vi "LoL Chat Front.vi"() -> ()   [LabVIEW 2011]
uses:
  <vilib>/addons/database/Connection.llb/DB Tools Open Connec (Path).vi
  <vilib>/addons/database/Connection.llb/Conn Execute.vi
  <vilib>/addons/database/Recordset.llb/Rec Fetch Recordset Data (R).vi
  <vilib>/Utility/file.llb/Write To Spreadsheet File (string).vi
  <vilib>/addons/database/NI_Database_API.lvlib
panel:
  out "Waveform Chart":i32[](graph)
  in  "Chat Time (minutes)":cluster{dbl, dbl}(slide)={0.0, 62.22222086588542} scale=0.0..150.0
  in  "Game Length (minutes)":cluster{dbl, dbl}(slide)={0.0, 62.22222086588542} scale=0.0..150.0
  in  "Word Length":cluster{dbl, dbl}(slide)={0.0, 8.585858585858587} scale=0.0..20.0
  out "Sorted Word Frequencies":string[][](array[string])
  in  "Save Results":bool
  out "SQL Query Command":string
  in  "Number of Entries":string="1000"
  in  "Game Outcome":string(combo)="Victory"
  in  "Scrollbar":i32(c297)
  in  "Tab Control 2":T1(tab)
  in  "Ashe":bool
  in  "Alistar":bool
  in  "Akali":bool
  in  "Ahri":bool
  in  "Aatrox":bool
  in  "Amumu":bool
  in  "Anivia":bool
  in  "Annie":bool
  in  "Darius":bool
  in  "Corki":bool
  in  "ChoGath":bool
  in  "Cassiopeia":bool
  in  "Caitlyn":bool
  in  "Braum":bool
  in  "Brand":bool
  in  "Blitzcrank":bool
  in  "Fiora":bool
  in  "Fiddlesticks":bool
  in  "Ezreal":bool
  in  "Evelynn":bool
  in  "Elise":bool
  in  "DrMundo":bool
  in  "Draven":bool
  in  "Diana":bool
  in  "Heimerdinger":bool
  in  "Hecarim":bool
  in  "Graves":bool
  in  "Gragas":bool
  in  "Garen":bool
  in  "Gangplank":bool
  in  "Galio":bool
  in  "Fizz":bool
  in  "Karthus":bool
  in  "Karma":bool
  in  "Jinx":bool
  in  "Jayce":bool
  in  "Jax":bool
  in  "JarvanIV":bool
  in  "Janna":bool
  in  "Irelia":bool
  in  "Lee sin":bool
  in  "Le Blanc":bool
  in  "Kog Maw":bool
  in  "Kha Zix":bool
  in  "Kennen":bool
  in  "Kayle":bool
  in  "Katarina":bool
  in  "Kassadin":bool
  in  "Blank Button 32":bool
  in  "Blank Button 31":bool
  in  "Blank Button 30":bool
  in  "Blank Button 29":bool
  in  "Blank Button 28":bool
  in  "Blank Button 27":bool
  in  "Blank Button 26":bool
  in  "Blank Button 25":bool
  in  "Blank Button 40":bool
  in  "Blank Button 39":bool
  in  "Blank Button 38":bool
  in  "Blank Button 37":bool
  in  "Blank Button 36":bool
  in  "Blank Button 35":bool
  in  "Blank Button 34":bool
  in  "Blank Button 33":bool
  in  "Blank Button 48":bool
  in  "Blank Button 47":bool
  in  "Blank Button 46":bool
  in  "Blank Button 45":bool
  in  "Blank Button 44":bool
  in  "Blank Button 43":bool
  in  "Blank Button 42":bool
  in  "Blank Button 41":bool
  in  "Blank Button 56":bool
  in  "Blank Button 55":bool
  in  "Blank Button 54":bool
  in  "Blank Button 53":bool
  in  "Blank Button 52":bool
  in  "Blank Button 51":bool
  in  "Blank Button 50":bool
  in  "Blank Button 49":bool
  in  "Blank Button 64":bool
  in  "Blank Button 63":bool
  in  "Blank Button 62":bool
  in  "Blank Button 61":bool
  in  "Blank Button 60":bool
  in  "Blank Button 59":bool
  in  "Blank Button 58":bool
  in  "Blank Button 57":bool
  in  "Blank Button 72":bool
  in  "Blank Button 71":bool
  in  "Blank Button 70":bool
  in  "Blank Button 69":bool
  in  "Blank Button 68":bool
  in  "Blank Button 67":bool
  in  "Blank Button 66":bool
  in  "Blank Button 65":bool
  in  "Blank Button 80":bool
  in  "Blank Button 79":bool
  in  "Blank Button 78":bool
  in  "Blank Button 77":bool
  in  "Blank Button 76":bool
  in  "Blank Button 75":bool
  in  "Blank Button 74":bool
  in  "Blank Button 73":bool
  in  "Blank Button 88":bool
  in  "Blank Button 87":bool
  in  "Blank Button 86":bool
  in  "Blank Button 85":bool
  in  "Blank Button 84":bool
  in  "Blank Button 83":bool
  in  "Blank Button 82":bool
  in  "Blank Button 81":bool
  in  "Blank Button 94":bool
  in  "Blank Button 93":bool
  in  "Blank Button 92":bool
  in  "Blank Button 91":bool
  in  "Blank Button 90":bool
  in  "Blank Button 89":bool
  in  "stop":bool
  in  "Search Champion":string="Anivia"
  out "Processed Entries":i32[](array[numeric])
  out "Full Entries":string[][](array[string])
  in  "connection information":path=path "C:/Users/Acer/Documents/LoL Chat Project/datalink.udl"
  # "Max"
  # "Min"
  # "Max"
  # "Min"
  # "Max"
  # "Min"
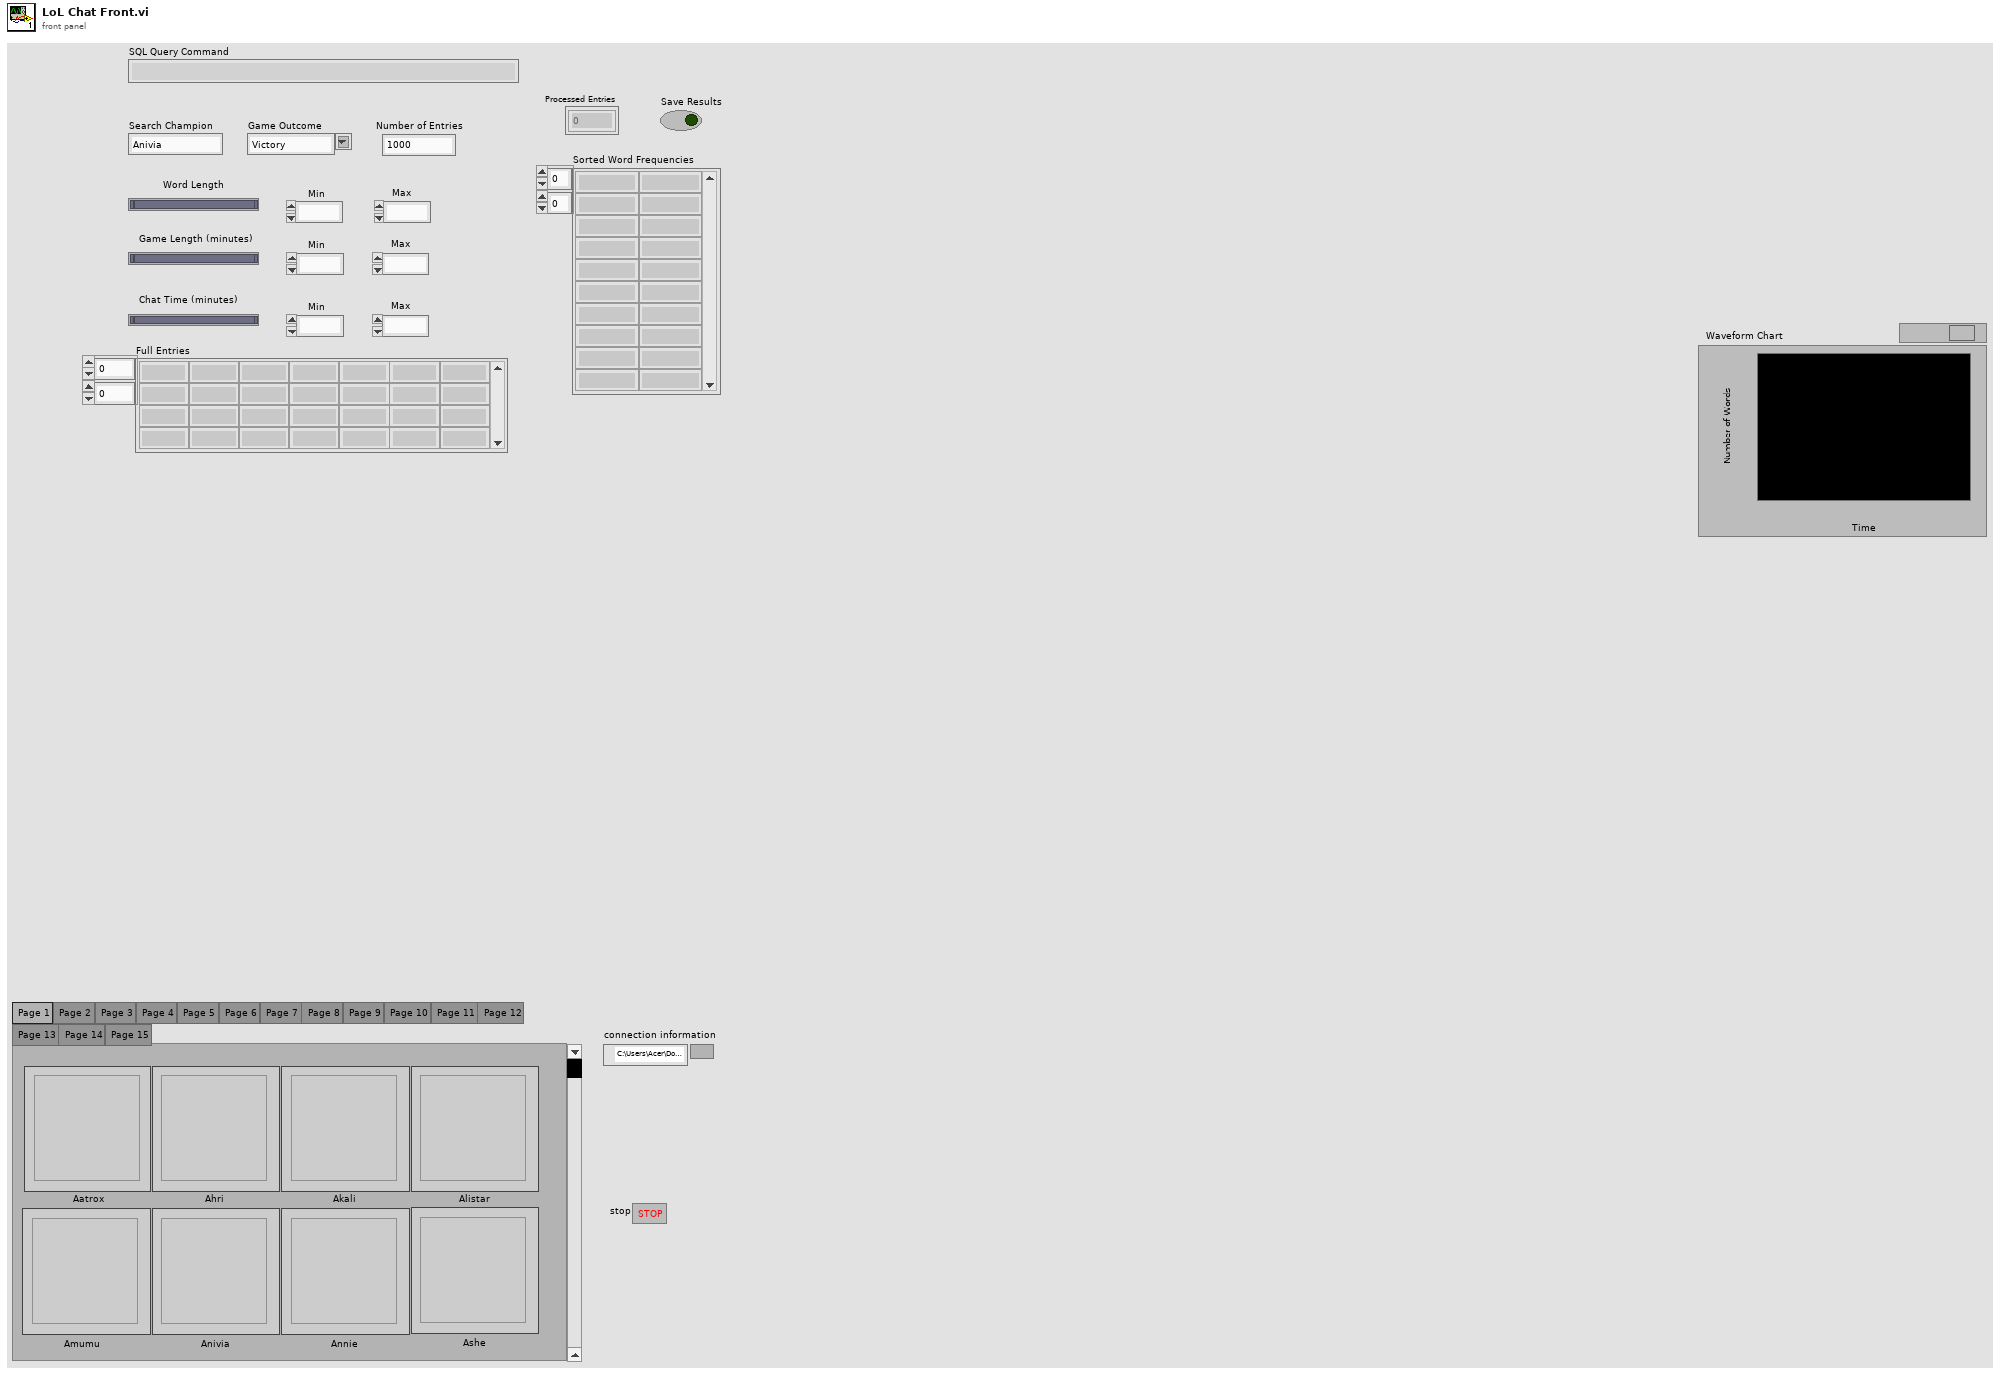
[diagram p1: front panel]
types:
  T1 = enum32{"Page 1", "Page 2", "Page 3", "Page 4", "Page 5", "Page 6", "Page 7", "Page 8", "Page 9", "Page 10", "Page 11", "Page 12", "Page 13", "Page 14", "Page 15"}
  T2 = typedef "NI_Database_API.lvlib/Conn ObjectReference.ctl" = refnum<k1>
  T3 = typedef "NI_Database_API.lvlib/Rec ObjectReference.ctl" = refnum<k1>
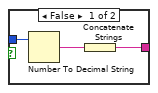
[diagram p3: hidden frame]
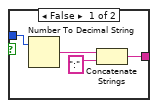
[diagram p4: hidden frame]
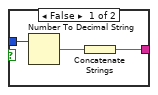
[diagram p5: hidden frame]
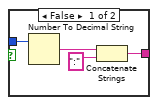
[diagram p6: hidden frame]
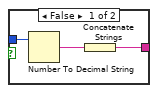
[diagram p7: hidden frame]
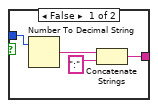
[diagram p8: hidden frame]
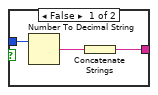
[diagram p9: hidden frame]
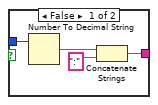
[diagram p10: hidden frame]
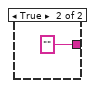
[diagram p12: hidden frame]
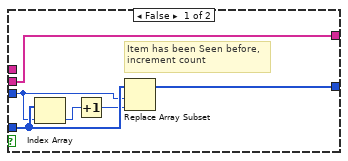
[diagram p13: hidden frame]
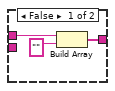
[diagram p14: hidden frame]
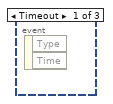
[diagram p15: hidden frame]
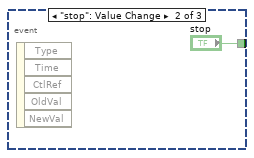
[diagram p16: hidden frame]
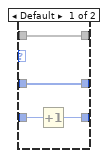
[diagram p18: hidden frame]
diagram:
  w12 = "#" ("string")
  w22 = 10 ("y")
  w15 = 60 ("x")
  w10 = "#" ("string")
  w27 = 10 ("y")
  (unwired) "SELECT TOP 1000 * FROM League_Data2 WHERE  TimeValue(TotalGameTime) BETWEEN #8:0:0# And #19:0:0# ; " ("SQL query")
  w36 = "#" ("string")
  w49 = 10 ("y")
  w39 = 60 ("x")
  w5 = " AND " ("string")
  w34 = "#" ("string")
  w55 = 10 ("y")
  (unwired) "SELECT * FROM League_Data2 WHERE Champion like '" ("SQL query")
  (unwired) "AND Result = '" ("string")
  w78 = i32[] []  # Count
  w77 = string[] []  # Elements Found
  (unwired) "SELECT * \n  FROM (SELECT * \n          FROM League_Data2 \n         WHERE Result = 'Victory')\nLIMIT 10 ;" ("SQL query")
  (unwired) "SELECT TOP 1000 * FROM League_Data2 WHERE  Result = 'Victory' ;" ("SQL query")
  (unwired) "SELECT Distinct ChatTime FROM League_Data2 ORDER BY ChatTime desc;" ("SQL query")
  n1 = disable-structure shown="Disabled" {
    frame Disabled {
      n2 = Index Array() -> (element=w104)  [unwired: 2 in]
      n3 = Initialize Array(w104, 0 ("Dimension Size")) -> (w105:void[])
      n4 = for {
        shift-right: [w112] -> _
        shift-left: w105 -> [w111]
        shift-right: [w109] -> _
        shift-left: 1 -> [w110]
        shift-right: [w107] -> _
        shift-left: i32[] [] -> [w108]
        n5 = Search 1D Array(1D array=w111) -> (index of element=w113:i32)  [unwired: 2 in]
        n6 = case shown="-1" w113 {
          tunnel: [w117 w122] -> w112
          tunnel: w111 -> [w117 w123]
          tunnel: w110 -> [w116 w119]
          tunnel: [w115 1] -> w109
          tunnel: w108 -> [w114 w120]
          tunnel: [w114 w118] -> w107
          frame Default {
            n7 = Increment(x=w116) -> (x+1=w115:i32)
          }
          frame -1 {
            n8 = Build Array (concatenate)(w123) -> (w122:void[])  [unwired: 1 in]
            n9 = Build Array (concatenate)(w120, w119) -> (w118:i32[])
          }
        }
      }
    }
    frame Enabled {
    }
  }
  n10 = disable-structure shown="Disabled" {
    frame Disabled {
      n11 = while {
        shift-right: _ -> [_]
        shift-left: string[] [] -> [_]
        stop <- w125 stop-if-true
        n12 = event shown="[2] \"Scrollbar\": Value Change" {
          selector: _ -> [_ _ _]
          dyn-events: _ -> [_ _ _]
          timeout: _ -> [_ _ _]
          tunnel: [_ "stop" _] -> w125
          event Timeout {
            n13 = event-data() -> ()  [unwired: 1 in, 2 out]
          }
          event "stop": Value Change {
            n14 = event-data() -> ()  [unwired: 1 in, 5 out]
          }
          event "Scrollbar": Value Change {
            n15 = event-data() -> ()  [unwired: 1 in, 5 out]
            n16 = property on="Tab Control 2" class="TabCtl (strict)"("Value"="Scrollbar") -> ()  [unwired: 2 in, 2 out]
          }
        }
        n17 = Wait Until Next ms Multiple(millisecond multiple=u32 100) -> ()  [unwired: 1 out]
      }
    }
    frame Enabled {
    }
  }
  n18 = Unbundle("Game Length (minutes)") -> (w59:dbl, w58:dbl)
  n19 = To Long Integer(number=w59) -> (32bit integer=w40:i32)
  n20 = To Long Integer(number=w58) -> (32bit integer=w43:i32)
  n21 = Quotient & Remainder(x=w40, y=w39) -> (x-y*floor(x/y)=w38:i32, floor(x/y)=w37:i32)
  n22 = Quotient & Remainder(x=w43, y=w39) -> (x-y*floor(x/y)=w42:i32, floor(x/y)=w41:i32)
  n23 = Less?(x=w38, y=w55) -> (x < y?=w54:bool)
  n24 = Less?(x=w37, y=w55) -> (x < y?=w57:bool)
  n25 = Less?(x=w42, y=w49) -> (x < y?=w48:bool)
  n26 = Less?(x=w41, y=w49) -> (x < y?=w51:bool)
  n27 = Equal?(x="Game Outcome", y="All") -> (x = y?=w71:bool)
  n28 = case shown="False" w71 {
    tunnel: [w129 "" ("string")] -> w67
    tunnel: "Game Outcome" -> [w132 _]
    frame False {
      n29 = Concatenate Strings("AND Result = '" ("string"), w132, "'" ("string")) -> (w129:string)
    }
    frame True {
    }
  }
  n30 = case shown="True" w54 {
    tunnel: w38 -> [w135 w140]
    tunnel: [w134 w137] -> w53
    frame False {
      n31 = Number To Decimal String(number=w135) -> (decimal integer string=w136:string)  [unwired: 1 in]
      n32 = Concatenate Strings(w136) -> (w134:string)
    }
    frame True {
      n33 = Number To Decimal String(number=w140) -> (decimal integer string=w139:string)  [unwired: 1 in]
      n34 = Concatenate Strings("0" ("string"), w139) -> (w137:string)
    }
  }
  n35 = case shown="True" w57 {
    tunnel: w37 -> [w142 w149]
    tunnel: [w141 w146] -> w56
    frame False {
      n36 = Number To Decimal String(number=w142) -> (decimal integer string=w144:string)  [unwired: 1 in]
      n37 = Concatenate Strings(w144, ":" ("string")) -> (w141:string)
    }
    frame True {
      n38 = Number To Decimal String(number=w149) -> (decimal integer string=w148:string)  [unwired: 1 in]
      n39 = Concatenate Strings("0" ("string"), w148, ":" ("string")) -> (w146:string)
    }
  }
  n40 = case shown="True" w48 {
    tunnel: w42 -> [w151 w156]
    tunnel: [w150 w153] -> w47
    frame False {
      n41 = Number To Decimal String(number=w151) -> (decimal integer string=w152:string)  [unwired: 1 in]
      n42 = Concatenate Strings(w152) -> (w150:string)
    }
    frame True {
      n43 = Number To Decimal String(number=w156) -> (decimal integer string=w155:string)  [unwired: 1 in]
      n44 = Concatenate Strings("0" ("string"), w155) -> (w153:string)
    }
  }
  n45 = case shown="True" w51 {
    tunnel: w41 -> [w158 w165]
    tunnel: [w157 w162] -> w50
    frame False {
      n46 = Number To Decimal String(number=w158) -> (decimal integer string=w160:string)  [unwired: 1 in]
      n47 = Concatenate Strings(w160, ":" ("string")) -> (w157:string)
    }
    frame True {
      n48 = Number To Decimal String(number=w165) -> (decimal integer string=w164:string)  [unwired: 1 in]
      n49 = Concatenate Strings("0" ("string"), w164, ":" ("string")) -> (w162:string)
    }
  }
  n50 = Unbundle("Chat Time (minutes)") -> (w31:dbl, w30:dbl)
  n51 = To Long Integer(number=w31) -> (32bit integer=w16:i32)
  n52 = To Long Integer(number=w30) -> (32bit integer=w19:i32)
  n53 = Quotient & Remainder(x=w16, y=w15) -> (x-y*floor(x/y)=w14:i32, floor(x/y)=w13:i32)
  n54 = Quotient & Remainder(x=w19, y=w15) -> (x-y*floor(x/y)=w18:i32, floor(x/y)=w17:i32)
  n55 = Less?(x=w14, y=w27) -> (x < y?=w26:bool)
  n56 = Less?(x=w13, y=w27) -> (x < y?=w29:bool)
  n57 = Less?(x=w18, y=w22) -> (x < y?=w21:bool)
  n58 = Less?(x=w17, y=w22) -> (x < y?=w24:bool)
  n59 = Concatenate Strings(w34, "" ("string"), w56, w53, w34) -> (w45:string)
  n60 = Concatenate Strings(w36, "" ("string"), w50, w47, w36) -> (w46:string)
  n61 = case shown="True" w26 {
    tunnel: w14 -> [w167 w172]
    tunnel: [w166 w169] -> w25
    frame False {
      n62 = Number To Decimal String(number=w167) -> (decimal integer string=w168:string)  [unwired: 1 in]
      n63 = Concatenate Strings(w168) -> (w166:string)
    }
    frame True {
      n64 = Number To Decimal String(number=w172) -> (decimal integer string=w171:string)  [unwired: 1 in]
      n65 = Concatenate Strings("0" ("string"), w171) -> (w169:string)
    }
  }
  n66 = case shown="True" w29 {
    tunnel: w13 -> [w174 w181]
    tunnel: [w173 w178] -> w28
    frame False {
      n67 = Number To Decimal String(number=w174) -> (decimal integer string=w176:string)  [unwired: 1 in]
      n68 = Concatenate Strings(w176, ":" ("string")) -> (w173:string)
    }
    frame True {
      n69 = Number To Decimal String(number=w181) -> (decimal integer string=w180:string)  [unwired: 1 in]
      n70 = Concatenate Strings("0" ("string"), w180, ":" ("string")) -> (w178:string)
    }
  }
  n71 = case shown="True" w21 {
    tunnel: w18 -> [w183 w188]
    tunnel: [w182 w185] -> w20
    frame False {
      n72 = Number To Decimal String(number=w183) -> (decimal integer string=w184:string)  [unwired: 1 in]
      n73 = Concatenate Strings(w184) -> (w182:string)
    }
    frame True {
      n74 = Number To Decimal String(number=w188) -> (decimal integer string=w187:string)  [unwired: 1 in]
      n75 = Concatenate Strings("0" ("string"), w187) -> (w185:string)
    }
  }
  n76 = case shown="True" w24 {
    tunnel: w17 -> [w190 w197]
    tunnel: [w189 w194] -> w23
    frame False {
      n77 = Number To Decimal String(number=w190) -> (decimal integer string=w192:string)  [unwired: 1 in]
      n78 = Concatenate Strings(w192, ":" ("string")) -> (w189:string)
    }
    frame True {
      n79 = Number To Decimal String(number=w197) -> (decimal integer string=w196:string)  [unwired: 1 in]
      n80 = Concatenate Strings("0" ("string"), w196, ":" ("string")) -> (w194:string)
    }
  }
  n81 = Concatenate Strings(w10, "" ("string"), w28, w25, w10) -> (w6:string)
  n82 = Concatenate Strings(w12, "" ("string"), w23, w20, w12) -> (w4:string)
  n83 = Concatenate Strings("SELECT TOP ", "Number of Entries", " * FROM League_Data3 WHERE Champion like '" ("SQL query"), "Search Champion", "%'", w67, "AND (TimeValue(TotalGameTime) BETWEEN " ("string"), w45, w5, w46, ")" ("string"), " AND (TimeValue(ChatTime) BETWEEN  " ("string"), w6, w5, w4, ");" ("string")) -> (w32:string)
  "SQL Query Command" <- w32
  n84 = call-poly <vilib>:"DB Tools Open Connection.vi"("prompt? (F)"=TRUE) -> ("connection reference"=w99:T2)  [unwired: 7 in, 1 out]
  n85 = call-poly <vilib>:"DB Tools Execute Query.vi"("SQL query"=w32, "connection reference"=w99) -> ("error out"=w100:errorcluster, "recordset reference"=w101:T3)  [unwired: 6 in]
  n86 = call-poly <vilib>:"DB Tools Fetch Recordset Data.vi"("error in (no error)"=w100, "recordset reference"=w101) -> ("recordset data"=w98:variant[][])  [unwired: 3 in, 2 out]
  n87 = for {
    tunnel: w98 -> [w199] mode=indexing
    tunnel: [w198] -> w94 mode=indexing
    n88 = for {
      tunnel: w199 -> [w201] mode=indexing
      tunnel: [w200] -> w198 mode=indexing
      n89 = Variant To Data(type="", Variant=w201) -> (data=w200:string)  [unwired: 1 in, 1 out]
    }
  }
  "Full Entries" <- w94
  n90 = Array Size(array=w94) -> (size(s)=→"Processed Entries":i32[])
  n91 = Index Array(array=w94, index (col)=4 ("disabled index (col)")) -> (element=w90:string[])  [unwired: 1 in]
  n92 = Index Array(array=w94, index (col)=6 ("disabled index (col)")) -> (element=w83:string[])  [unwired: 1 in]
  n93 = To Lower Case(string=w83) -> (all lower case string=w82:string[])
  n94 = for {
    tunnel: w90 -> [w206] mode=indexing
    tunnel: w82 -> [w210] mode=indexing
    shift-right: [w203] -> w79
    shift-left: string[][] [] ("array type (2D Dbl)") -> [w205]
    n95 = Spreadsheet String To Array(delimiter (Tab)=" ", format string="%s", spreadsheet string=w210, array type (2D Dbl)=string[] []) -> (array=w208:string[])
    n96 = for {
      tunnel: w208 -> [w221] mode=indexing
      tunnel: w206 -> [w223]
      tunnel: [w222] -> w204 mode=indexing
      n97 = Unbundle("Word Length") -> (w213:dbl, w215:dbl)
      n98 = To Long Integer(number=w215) -> (32bit integer=w214:i32)
      n99 = To Long Integer(number=w213) -> (32bit integer=w212:i32)
      n100 = String Length(string=w221) -> (length=w220:i32)
      n101 = Less?(x=w220, y=w214) -> (x < y?=w218:bool)
      n102 = Less?(x=w212, y=w220) -> (x < y?=w219:bool)
      n103 = And(x=w218, y=w219) -> (x .and. y?=w217:bool)
      n104 = case shown="True" w217 {
        tunnel: w223 -> [w226 w229]
        tunnel: [w224 w228] -> w222
        tunnel: w221 -> [_ w227]
        frame False {
          n105 = Build Array(w226, "" ("element")) -> (w224:string[])
        }
        frame True {
          n106 = Build Array(w229, w227) -> (w228:string[])
        }
      }
    }
    n107 = Insert Into Array(array=w205, new element=w204) -> (w203:string[][])  [unwired: 2 in]
  }
  n108 = Index Array(array=w79, index (col)=1 ("disabled index (col)")) -> (element=w87:string[])  [unwired: 1 in]
  n109 = Sort 1D Array(array=w87) -> (sorted array=w74:string[])
  n110 = for {
    tunnel: w74 -> [w234] mode=indexing
    shift-right: [w233] -> w75
    shift-left: w77 -> [w235]
    shift-right: [w231] -> w76
    shift-left: w78 -> [w232]
    # "-1 means the item is not found"
    # "check if item has been seen\nbefore"
    n111 = Search 1D Array(1D array=w235, element=w234) -> (index of element=w230:i32)  [unwired: 1 in]
    n112 = Equal?(x=w230, y=-1) -> (x = y?=w236:bool)
    n113 = case shown="True" w236 {
      tunnel: w235 -> [w243 w249]
      tunnel: w234 -> [_ w248]
      tunnel: [w243 w247] -> w233
      tunnel: w232 -> [w242 w246]
      tunnel: [w238 w244] -> w231
      tunnel: w230 -> [w241 _]
      frame False {
        # "Item has been Seen before,\nincrement count"
        n114 = Index Array(array=w242, index=w241) -> (element=w239:i32)
        n115 = Increment(x=w239) -> (x+1=w240:i32)
        n116 = Replace Array Subset(array=w242, new element=w240, index=w241) -> (w238:i32[])
      }
      frame True {
        # "Add new item to array and start\ncount at 1."
        n117 = Build Array (concatenate)(w249, w248) -> (w247:string[])
        n118 = Build Array (concatenate)(w246, 1) -> (w244:i32[])
      }
    }
  }
  n119 = Number To Decimal String(number=w76) -> (decimal integer string=w84:string[])  [unwired: 1 in]
  n120 = Build Array(w75, w84) -> (w81:string[][])
  n121 = Transpose 2D Array(2D array=w81) -> (transposed array=w80:string[][])
  n122 = call "2d_Array_sortSimplified.vi"("Column to Sort on"=1, "2D Input Array"=w80, "Sort numerically"=TRUE) -> ("2D Ouput Array"=w61:string[][])
  n123 = Array Size(array=w61) -> (size(s)=w66:i32[])
  n124 = Index Array(array=w66) -> (element=w64:i32)  [unwired: 1 in]
  n125 = case shown="True" "Save Results" {
    tunnel: w61 -> [_ w250]
    frame False {
    }
    frame True {
      n126 = call-poly <vilib>:"Write To Spreadsheet File.vi"("2D data"=w250) -> ()  [unwired: 7 in, 1 out]
    }
  }
  n127 = Decrement(x=w64) -> (x-1=w62:i32)
  n128 = Logical Shift(y=i8 -1, x=w64) -> (x << y=w65:i32)
  n129 = for {
    N: w65 -> [_]
    shift-right: [w257] -> w2
    shift-left: w61 -> [w256]
    tunnel: w62 -> [w253]
    i -> [w252]
    n130 = Subtract(x=w253, y=w252) -> (x-y=w251:i32)
    n131 = Index Array(array=w256, index (row) #1=w252, index (row) #2=w251) -> (element #1=w254:string[], element #2=w255:string[])  [unwired: 2 in]
    n132 = Replace Array Subset(array=w256, new element #1=w255, index (row) #1=w252, new element #2=w254, index (row) #2=w251) -> (w257:string[][])  [unwired: 2 in]
  }
  "Sorted Word Frequencies" <- w2
  n133 = disable-structure shown="Disabled" {
    disable-tunnel: w2 -> [w264 _]
    frame Disabled {
      n134 = Index Array(array=w264, index (col)=1 ("disabled index (col)")) -> (element=w262:string[])  [unwired: 1 in]
      n135 = Array Subset(array=w262, index=1, length=10) -> (w259:string[])
      n136 = Decimal String To Number(string=w259) -> (number=→"Waveform Chart":i32[])  [unwired: 2 in, 1 out]
    }
    frame Enabled {
    }
  }
